vi "9.2.-SubVI Escala de Grises y Binarizado Imagen.vi"(11 "Ruta de Imagen (.bmp)":path) -> (2 "Array de la imagen con escala de grises":u32[][](array[numeric]), 3 "Figura":picture)   [LabVIEW 2020]
panel:
  # "Visión Artificial - Firma de Figuras\nDiego Cervantes Rodríguez\ndicer0.com"
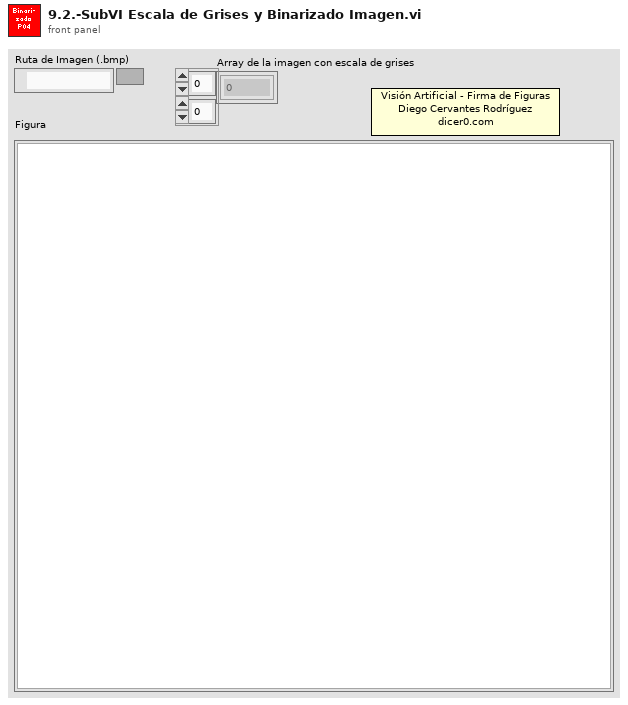
[diagram p1: front panel]
types:
  T1 = typedef "imagedata.ctl" = cluster{"image type":i32, "image depth":i32, "image":u8[], "mask":u8[], "colors":u32[], "Rectangle":cluster{"left":i16, "top":i16, "right":i16, "bottom":i16}}
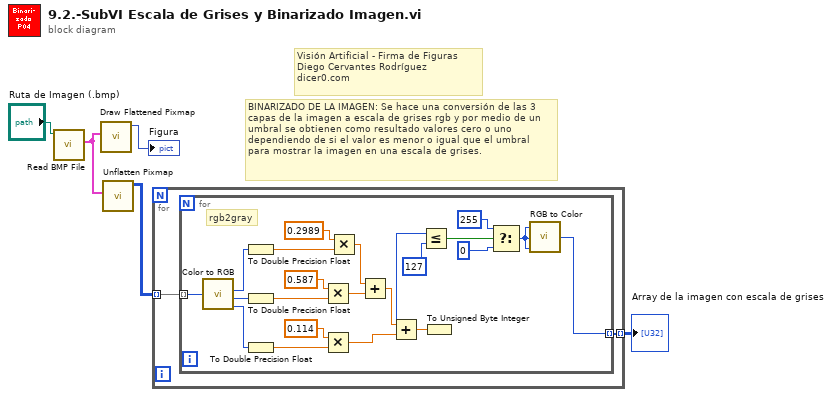
[diagram p0: block diagram]
diagram:
  # "Visión Artificial - Firma de Figuras\nDiego Cervantes Rodríguez\ndicer0.com"
  # "BINARIZADO DE LA IMAGEN: Se hace una conversión de las 3 capas de la imagen a escala de grises rgb y por medio de un umbral se obtienen como resultado valores cero o uno dependiendo de si el valor es menor o igual que el umbral  para mostrar la imagen en una escala de grises."
  n1 = call <vilib>:"Read BMP File.vi"("path to BMP file"="Ruta de Imagen (.bmp)") -> ("image data"=w2:T1)  [unwired: 8 in, 2 out]
  n2 = call <vilib>:"Draw Flattened Pixmap.vi"("image data"=w2) -> ("new picture"=→"Figura":picture)  [unwired: 8 in]
  n3 = call <vilib>:"Unflatten Pixmap.vi"("image data"=w2) -> ("24-bit pixmap"=w3:u32[][])  [unwired: 4 in, 6 out]
  n4 = for {
    tunnel: w3 -> [w7] mode=indexing
    tunnel: [w6] -> w5 mode=indexing
    n5 = for {
      tunnel: w7 -> [w15] mode=indexing
      tunnel: [w8] -> w6 mode=indexing
      # "rgb2gray"
      n6 = call <vilib>:"Color to RGB.vi"("Color"=w15) -> ("R"=w28:u8, "G"=w27:u8, "B"=w26:u8)  [unwired: 1 out]
      n7 = To Double Precision Float(number=w28) -> (double precision float=w19:dbl)
      n8 = To Double Precision Float(number=w27) -> (double precision float=w20:dbl)
      n9 = To Double Precision Float(number=w26) -> (double precision float=w21:dbl)
      n10 = Multiply(x=0.587, y=w20) -> (x*y=w22:dbl)
      n11 = Multiply(x=0.114, y=w21) -> (x*y=w25:dbl)
      n12 = Multiply(x=0.2989, y=w19) -> (x*y=w23:dbl)
      n13 = Add(x=w23, y=w22) -> (x+y=w24:dbl)
      n14 = Add(x=w24, y=w25) -> (x+y=w29:dbl)
      n15 = To Unsigned Byte Integer(number=w29) -> (unsigned 8bit integer=w11:u8)
      n16 = Less Or Equal?(x=w11, y=u8 127) -> (x <= y?=w14:bool)
      n17 = Select(t=u8 255, s=w14, f=u8 0) -> (s? t:f=w9:u8)
      n18 = call <vilib>:"RGB to Color.vi"("B"=w9, "G"=w9, "R"=w9) -> ("Color"=w8:u32)
    }
  }
  "Array de la imagen con escala de grises" <- w5
